vi "1DTurnMain.vi"() -> ()   [LabVIEW 2017]
panel:
  in  "Gains":T1={"Gains"={"FFV"=0.0021, "FFA"=0.0001, "Vel PID"={"P"=0.002, "I"=0.0, "D"=0.0}}, "Pos PID"={"P"=0.002, "I"=0.0, "D"=0.0}, "MinVoltage"=0.0} {"Pos PID"."D" format="%.3f"; "Pos PID"."I" format="%.3f"; "Pos PID"."P" format="%.3f"; "Gains"."Vel PID"."D" format="%.3f"; "Gains"."Vel PID"."I" format="%.3f"; "Gains"."Vel PID"."P" format="%.3f"}
  out "Power":dbl(graph)
  in  "StartAngle":dbl
  out "Done?":bool
  out "Vel":cluster{"Output":dbl, "dx/dt":dbl}(graph)={"Output"=0.0, "dx/dt"=-2.5707427177340247}
  out "Pos":cluster{"Distance":dbl, "CurrentAngle":dbl}(graph)
  in  "Config":T2={"Gear Reduction"=15.0, "Wheel Radius (m)"=0.076, "# Motors"=6, "coeff of friction"=0.1, "Mass (kg)"=50.0, "Motor"={"Ke (V)"=0.0183, "R (ohms)"=0.09, "KT (Nm/A)"=0.0183, "Tf (Nm)"=0.4}}
  in  "TargetAngle":dbl=90.0
  in  "MaxVel":dbl=300.0
  in  "MaxAccel":dbl=400.0
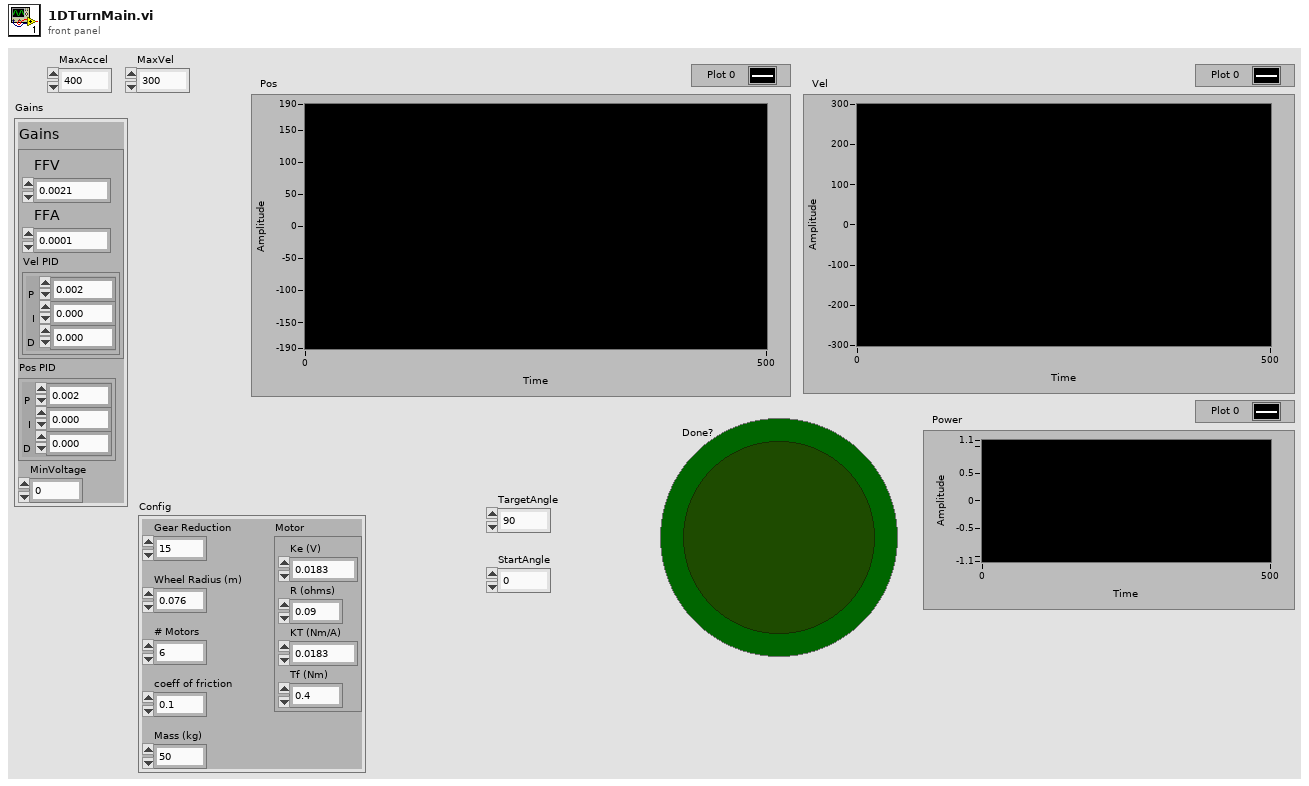
[diagram p1: front panel]
types:
  T1 = cluster{"Gains":cluster{"FFV":dbl, "FFA":dbl, "Vel PID":cluster{"P":dbl, "I":dbl, "D":dbl}}, "Pos PID":cluster{"P":dbl, "I":dbl, "D":dbl}, "MinVoltage":dbl}
  T2 = cluster{"Gear Reduction":dbl, "Wheel Radius (m)":dbl, "# Motors":u32, "coeff of friction":dbl, "Mass (kg)":dbl, "Motor":cluster{"Ke (V)":dbl, "R (ohms)":dbl, "KT (Nm/A)":dbl, "Tf (Nm)":dbl}}
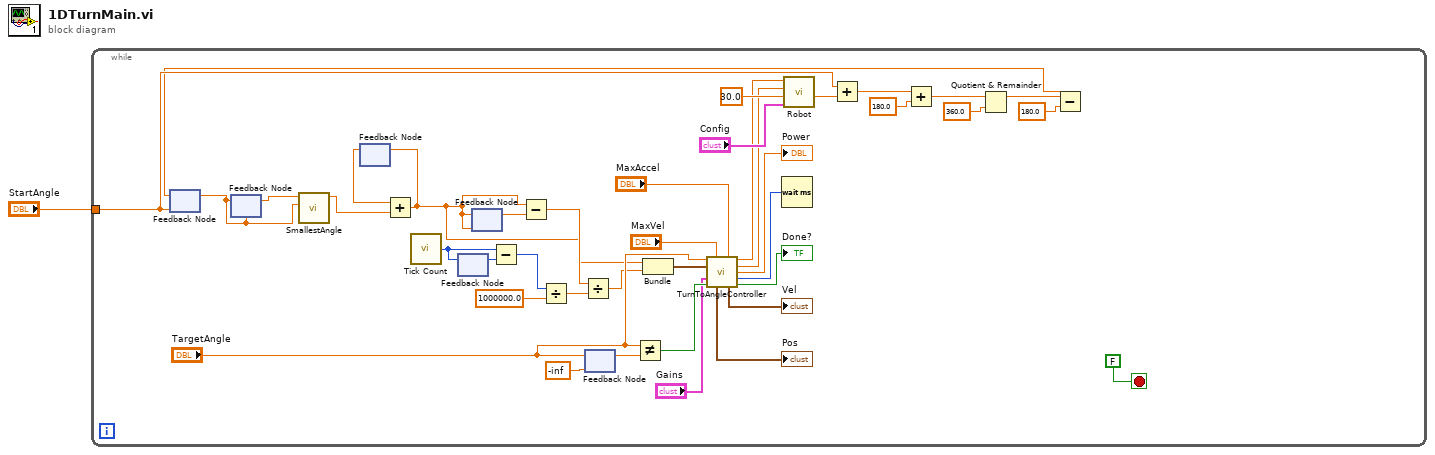
[diagram p0: block diagram]
diagram:
  n1 = while {
    tunnel: "StartAngle" -> [w19]
    stop <- FALSE stop-if-true
    n2 = feedback #1(w19) -> (w4:dbl)
    n3 = feedback-in #2(w4) -> ()
    n4 = feedback #2(w4) -> (w5:dbl)
    n5 = call "SmallestAngle.vi"("Angle B"=w4, "Angle A"=w5) -> ("Smallest A to B"=w6:dbl)  [unwired: 9 in]
    n6 = feedback #3() -> (w8:dbl)  [unwired: 1 in]
    n7 = Add(x=w8, y=w6) -> (x+y=w2:dbl)
    n8 = feedback-in #3(w2) -> ()
    n9 = call "Tick Count"() -> ("Tick Count(uSec)"=w11:u32)
    n10 = feedback #4() -> (w13:u32)  [unwired: 1 in]
    n11 = feedback-in #4(w11) -> ()
    n12 = feedback-in #5(w2) -> ()
    n13 = feedback #5(w2) -> (w15:dbl)
    n14 = Subtract(x=w11, y=w13) -> (x-y=w12:u32)
    n15 = Subtract(x=w2, y=w15) -> (x-y=w17:dbl)
    n16 = Divide(x=w12, y=1000000.0) -> (x/y=w9:dbl)
    n17 = Divide(x=w17, y=w9) -> (x/y=w14:dbl)
    n18 = feedback-in #6("TargetAngle") -> ()
    n19 = feedback #6(-inf ("TargetAngle")) -> (w29:dbl)
    n20 = Not Equal?(x="TargetAngle", y=w29) -> (x != y?=w28:bool)
    n21 = Bundle(w2, w14) -> (w16:cluster{dbl, dbl})  [unwired: 1 in]
    n22 = call "TurnToAngleController.vi"("TargetAngle"="TargetAngle", "MaxVel"="MaxVel", "MaxAccel"="MaxAccel", "Robot"=w16, "Gains"="Gains", "Reset"=w28) -> ("LeftPower"=w34:dbl, "RightPower"=w33:dbl, "Power"=→"Power":dbl, "Delay"=w38:u32, "Pos"=→"Pos":cluster{"Distance":dbl, "CurrentAngle":dbl}, "VelGraph"=→"Vel":cluster{"Output":dbl, "dx/dt":dbl}, "Done"=→"Done?":bool)  [unwired: 3 in]
    n23 = Wait (ms)(milliseconds to wait=w38) -> ()  [unwired: 1 out]
    n24 = call "Robot.vi"("Config"="Config", "WheelBase"=30.0, "Right Value"=w33, "Left Value"=w34) -> ("Angle"=w21:dbl)  [unwired: 5 in, 2 out]
    n25 = Add(x=w19, y=w21) -> (x+y=w20:dbl)
    n26 = Add(x=w20, y=180.0) -> (x+y=w25:dbl)
    n27 = Quotient & Remainder(x=w25, y=360.0) -> (x-y*floor(x/y)=w23:dbl)  [unwired: 1 out]
    n28 = Subtract(x=w23, y=180.0) -> (x-y=w7:dbl)
    n29 = feedback-in #1(w7) -> ()
  }
